vi "Write Delimiters.vi"(8 "Error In":errorcluster, 10 "Delimiters":T1={"Close"="}}", "Open"="{{"}, 11 "Node In":refnum<class "Abstract.lvclass">) -> (0 "Error Out":errorcluster, 3 "Node Out":refnum<class "Abstract.lvclass">)   [LabVIEW 2018, in "Toolkit.lvlib" / "Nodes.lvlib" / "Abstract.lvclass"]
doc: "Sets the opening and closing components that surround, or delimit, a Mustache tag."
uses:
  Abstract.lvclass
  Type Definitions/Delimiters.ctl
  Abstract.lvclass/Abstract.ctl
  Toolkit.lvlib
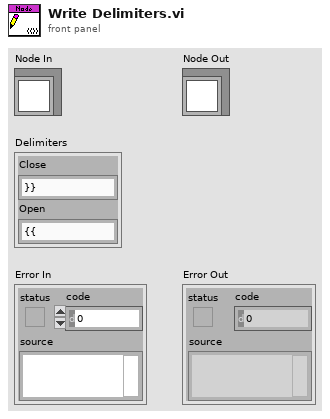
[diagram p1: front panel]
types:
  T1 = typedef "Toolkit.lvlib/Delimiters.ctl" = cluster{"Close":string, "Open":string}
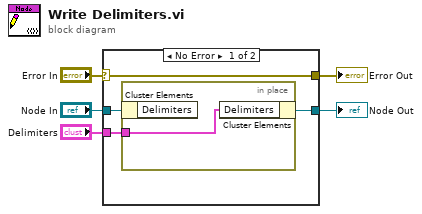
[diagram p0: block diagram]
diagram:
  n1 = case shown="No Error" "Error In" {
    selector: "Error In" -> [w9 w11]
    tunnel: [w9 w11] -> w4
    tunnel: [w7 w12] -> w2
    tunnel: "Node In" -> [w8 w12]
    tunnel: "Delimiters" -> [w6 _]
    frame No Error {
      n2 = in-place {
        in-place-border: w6 -> [w10]
        n3 = in-place-cluster #1(w8) -> ()  [unwired: 1 out]
        n4 = in-place-cluster #1("Delimiters"=w10) -> (w7:refnum<class "Abstract.lvclass">)
      }
    }
    frame Error {
    }
  }
  "Error Out" <- w4
  "Node Out" <- w2
